vi "555集成定时器组成多谐振荡器.vi"() -> ()   [LabVIEW 2018]
panel:
  in  "R1":dbl
  out "V":dbl
  out "波形图表":cluster{"V":dbl, i16}(graph)
  out "毫秒计时值 2":u32
  out "毫秒计时值":u32
  in  "C":dbl
  in  "R2":dbl
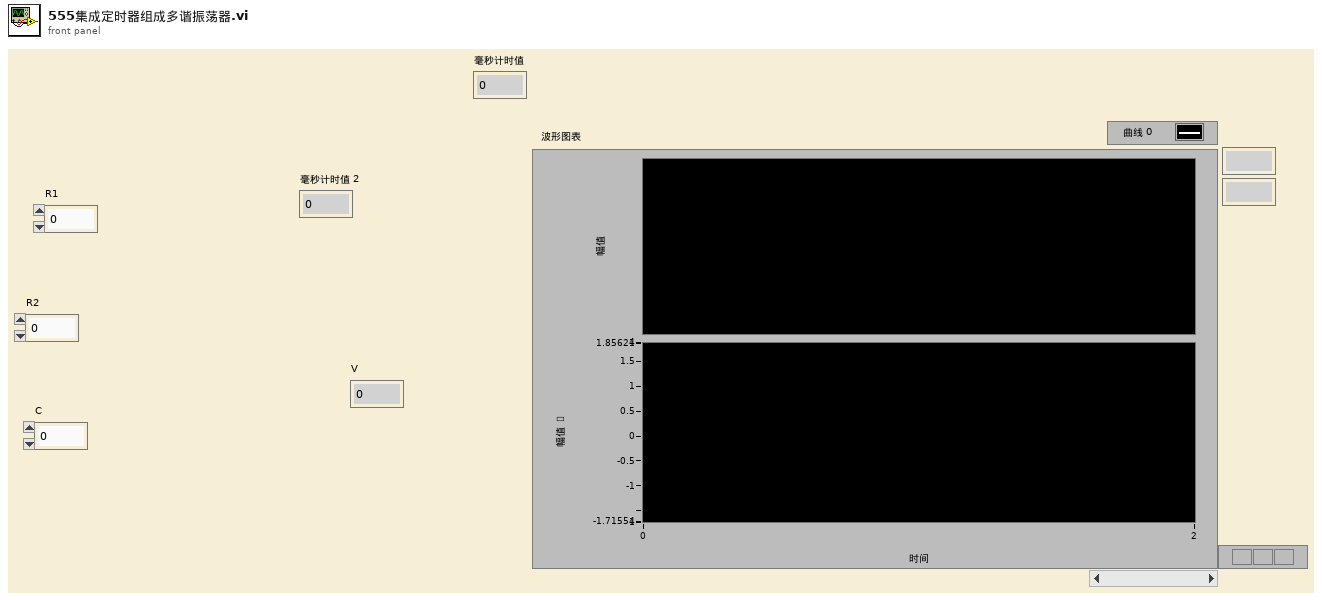
[diagram p1: front panel]
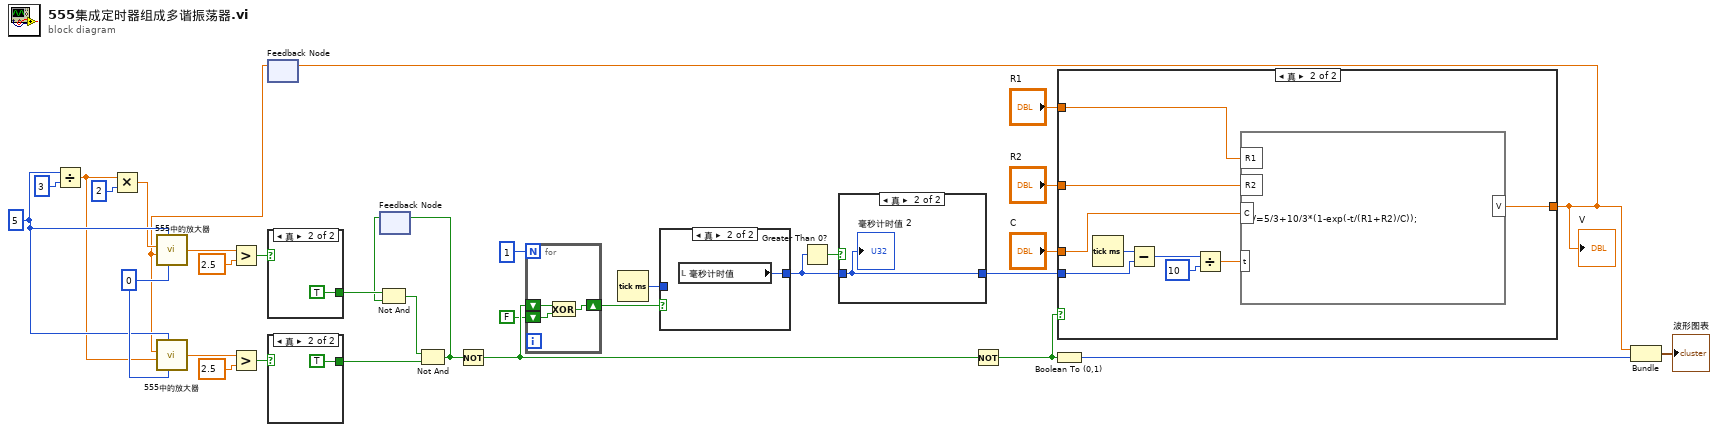
[diagram p0: block diagram]
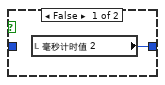
[diagram p2: hidden frame]
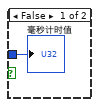
[diagram p3: hidden frame]
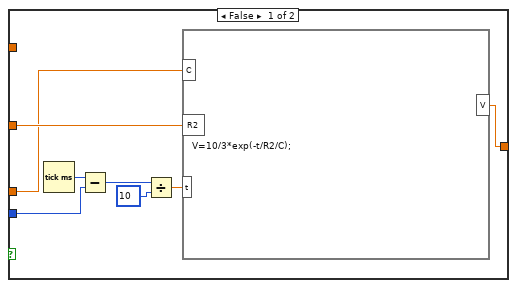
[diagram p4: hidden frame]
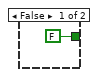
[diagram p5: hidden frame]
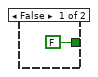
[diagram p6: hidden frame]
diagram:
  w33 = 0
  w21 = 5
  n1 = Divide(x=w21, y=3) -> (x/y=w19:dbl)
  n2 = Multiply(x=w19, y=2) -> (x*y=w18:dbl)
  n3 = feedback #1() -> (w7:dbl)  [unwired: 1 in]
  n4 = call "555中的放大器.vi"("VCC"=w21, "IN+"=w18, "IN--"=w7, "--VCC"=w33) -> ("OUT"=w32:dbl)  [unwired: 4 in]
  n5 = call "555中的放大器.vi"("VCC"=w21, "IN+"=w7, "IN--"=w19, "--VCC"=w33) -> ("OUT"=w27:dbl)  [unwired: 4 in]
  n6 = Greater?(x=w32, y=2.5) -> (0:w30:bool)
  n7 = Greater?(x=w27, y=2.5) -> (0:w28:bool)
  n8 = case shown="真" w30 {
    tunnel: [FALSE TRUE] -> w26
    frame False {
    }
    frame True {
    }
  }
  n9 = case shown="真" w28 {
    tunnel: [FALSE TRUE] -> w25
    frame False {
    }
    frame True {
    }
  }
  n10 = feedback #2() -> (w23:bool)  [unwired: 1 in]
  n11 = Not And(1:w23, 2:w26) -> (0:w24:bool)
  n12 = Not And(1:w25, 2:w24) -> (0:w22:bool)
  n13 = feedback-in #2(w22) -> ()
  n14 = Not(x=w22) -> (.not. x?=w16:bool)
  n15 = for {
    N: 1 -> [_]
    shift-right: [w38] -> w12
    shift-left: w16 -> [w40]
    shift-left: FALSE -> [w39]
    n16 = Exclusive Or(1:w39, 2:w40) -> (0:w38:bool)
  }
  n17 = Tick Count (ms)() -> (millisecond timer value=w13:u32)
  n18 = case shown="真" w12 {
    tunnel: w13 -> [w41 _]
    tunnel: [_ w42] -> w10
    frame False {
      "毫秒计时值" <- w41
    }
    frame True {
      n19 = local read "毫秒计时值"() -> (w42:u32)
    }
  }
  n20 = Greater Than 0?(x=w10) -> (x > 0?=w11:bool)
  n21 = case shown="真" w11 {
    tunnel: w10 -> [_ w44]
    tunnel: [w43 w44] -> w9
    frame False {
      n22 = local read "毫秒计时值 2"() -> (w43:u32)
    }
    frame True {
      "毫秒计时值 2" <- w44
    }
  }
  n23 = Not(x=w16) -> (.not. x?=w6:bool)
  n24 = Boolean To (0,1)(Boolean=w6) -> (0, 1=w4:i16)
  n25 = case shown="真" w6 {
    tunnel: w9 -> [w51 w60]
    tunnel: "R1" -> [_ w54]
    tunnel: "R2" -> [w48 w55]
    tunnel: "C" -> [w46 w56]
    tunnel: [w45 w53] -> w5
    frame False {
      n26 = Tick Count (ms)() -> (millisecond timer value=w52:u32)
      n27 = Subtract(x=w52, y=w51) -> (x-y=w50:u32)
      n28 = Divide(x=w50, y=u32 10) -> (x/y=w47:dbl)
      n29 = formula code="V=10/3*exp(-t/R2/C);"("t"=w47, "R2"=w48, "C"=w46) -> ("V"=w45:dbl)
    }
    frame True {
      n30 = Tick Count (ms)() -> (millisecond timer value=w61:u32)
      n31 = Subtract(x=w61, y=w60) -> (x-y=w59:u32)
      n32 = Divide(x=w59, y=u32 10) -> (x/y=w57:dbl)
      n33 = formula code="V=5/3+10/3*(1-exp(-t/(R1+R2)/C));"("t"=w57, "R2"=w55, "C"=w56, "R1"=w54) -> ("V"=w53:dbl)
    }
  }
  "V" <- w5
  n34 = feedback-in #1(w5) -> ()
  n35 = Bundle("V"=w5, w4) -> (→"波形图表":cluster{"V":dbl, i16})  [unwired: 1 in]
